vi "OverviewGUI.vi"() -> ()   [LabVIEW 2011]
panel:
  in  "End":bool
  in  "Registerkarte":enum32{"Goto", "Load file", "Load mem", "debug"}(tab)=enum."Load file"
  in  "pos [m]":cluster{dbl, dbl} {"?" format="%#_6p"; "?" format="%#_6p"}
  in  "Goto":bool
  in  "max":cluster{dbl, dbl}={0.066325, 0.044039}
  in  "min":cluster{dbl, dbl}={0.053456, 0.031964}
  in  "Load":bool
  in  "Single tiff":path
  in  "Val2":sgl=4095.0
  in  "Val1":sgl
  in  "Mode":enum16{"Min, Max", "Low%,High%", "Full"}(ring)
  in  "OK-Schaltfläche":bool
  in  "exp.":string="experiment700"
  in  "Pixels":dbl=1000000.0
  in  "Clear":bool
  in  "Add":bool
  in  "Number":u16
  in  "Start":u16
  in  "Calculate":bool
  in  "IMAQs":i32[](array[numeric])
  in  "Transform (Center first)":T1={"Center"={0.0, 0.0}, "Rotate (rad)"=0.0, "MirrorY"=FALSE, "Scale"=1.0}
  out "Image":T2(plugin-control)
  # "known corner coordinates"
  # "left down"
  # "right up"
  # "135CCD"
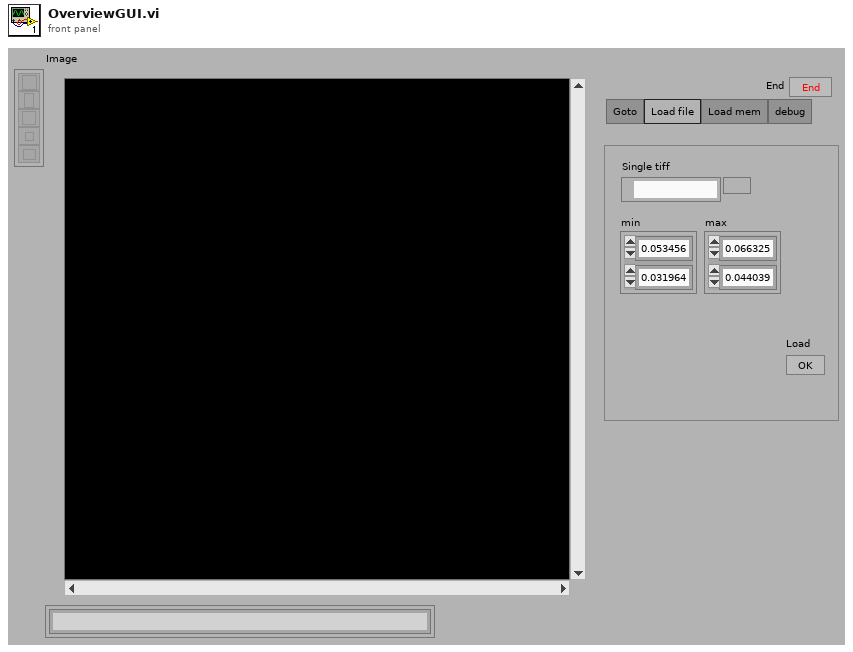
[diagram p1: front panel]
types:
  T1 = cluster{"Center":cluster{dbl, dbl}, "Rotate (rad)":dbl, "MirrorY":bool, "Scale":dbl}
  T2 = typedef "IMAQ Image.ctl" = refnum<image>
  T3 = typedef "Image Type" = u32
  T4 = enum16{"None/#Datasets", "Clear", "TagValueOf#", "AddValues", "ReadValue", "ChangeValue", "Get all"}
  T5 = enum16{"status", "createIMAQ", "getIMAQ", "getNumber", "deleteIMAQ", "deleteAll", "MemoryUsage", "GetAccess", "DecreaseAccess", "ActualIndex", "ElementToNumber"}
  T6 = enum16{"status", "saveMeta", "getMeta", "deleteMeta", "deleteAll", "MemoryUsage"}
  T7 = cluster{"Global Rectangle":i32[], "Contours":cluster{"Contour Type":u32, "ROI Type":u32, "Points":i32[]}[]}
  T8 = typedef "IMAQ Point" = cluster{"X":sgl, "Y":sgl}
  T9 = cluster{cluster{dbl, dbl}, dbl, bool, "pixel/size":dbl}
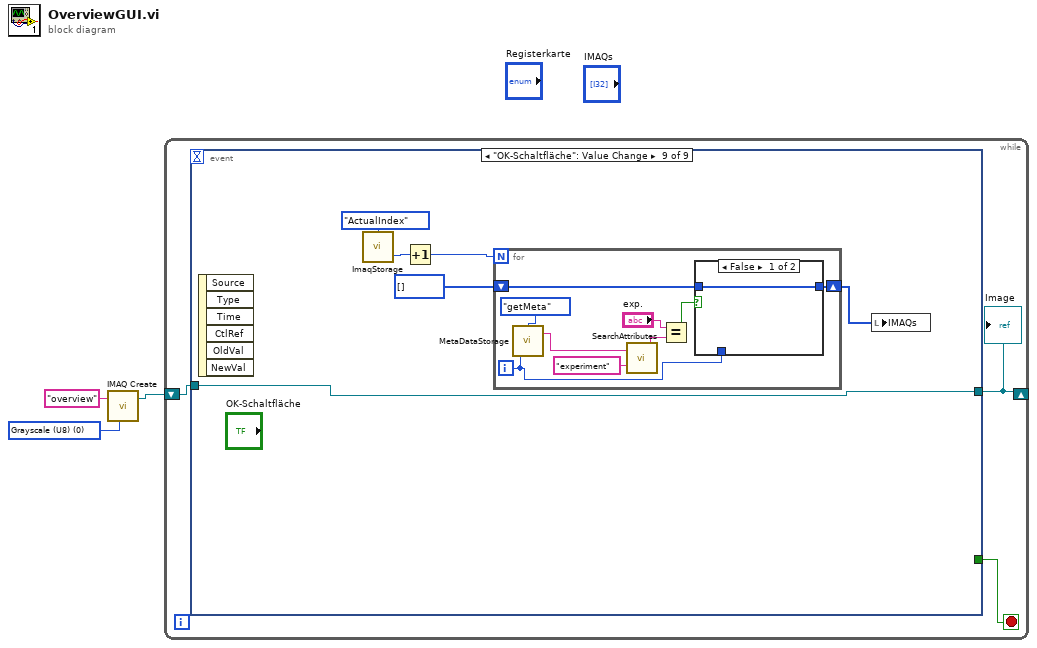
[diagram p0: block diagram]
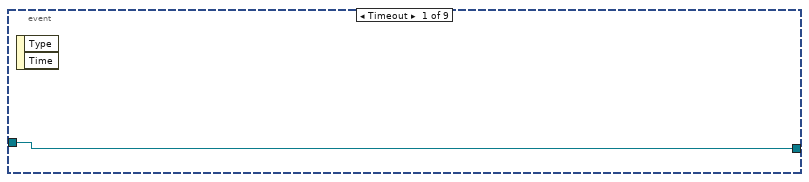
[diagram p2: hidden frame]
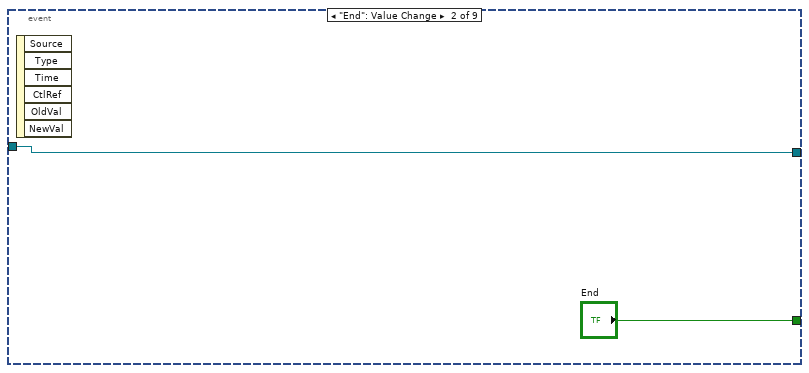
[diagram p3: hidden frame]
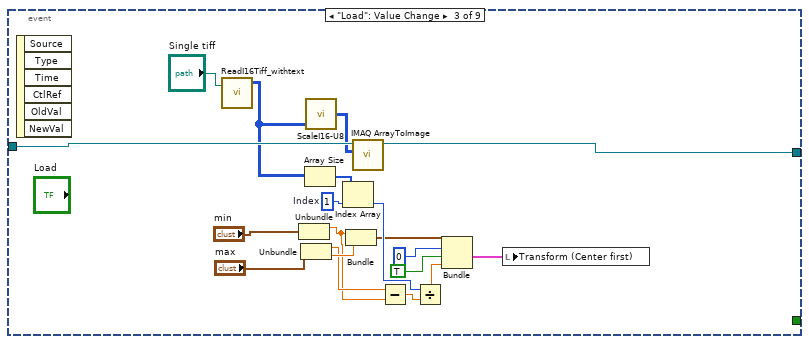
[diagram p4: hidden frame]
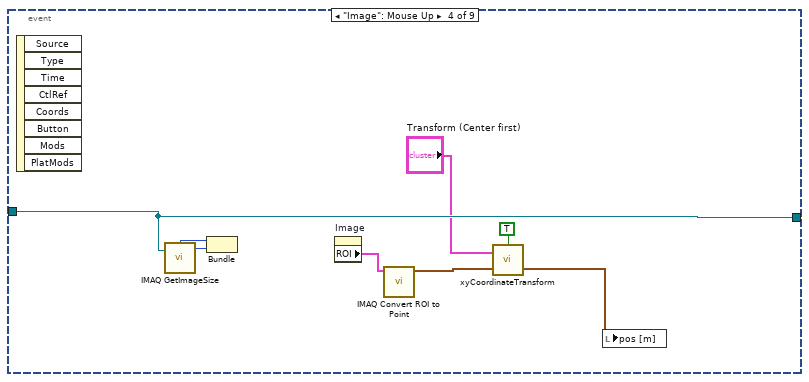
[diagram p5: hidden frame]
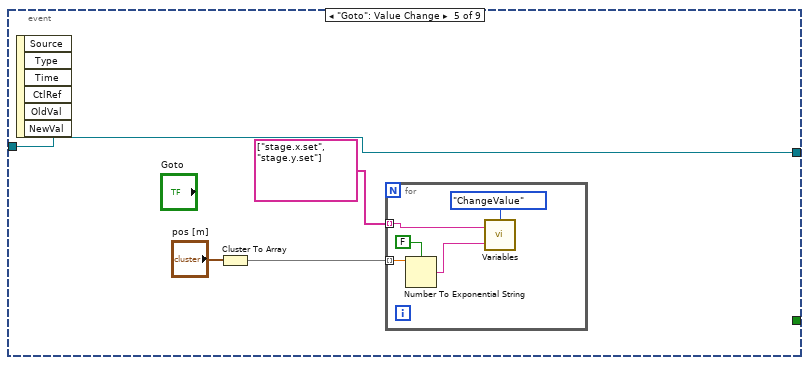
[diagram p6: hidden frame]
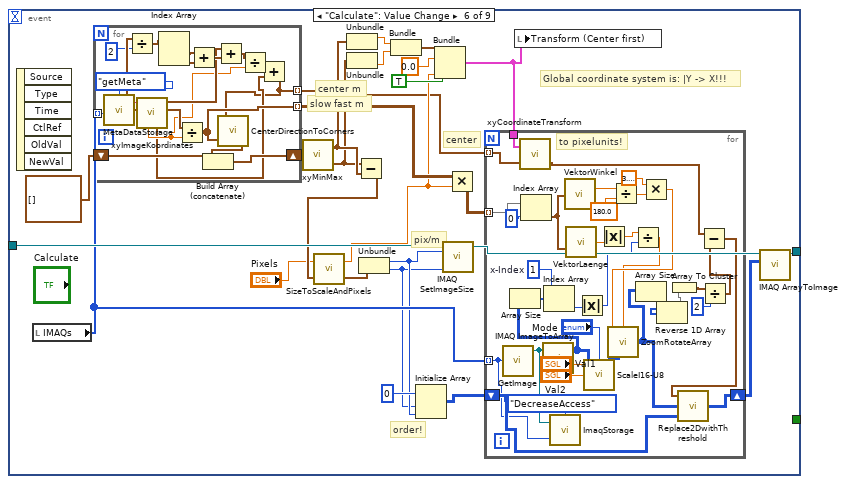
[diagram p7: hidden frame]
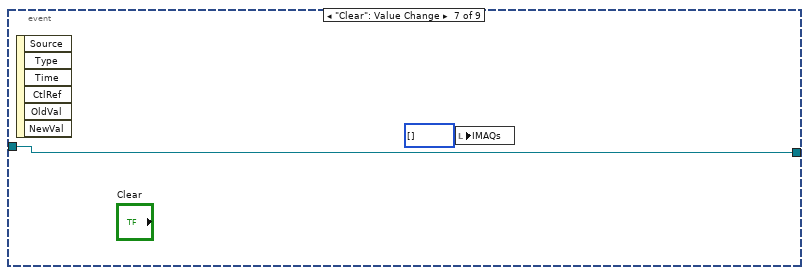
[diagram p8: hidden frame]
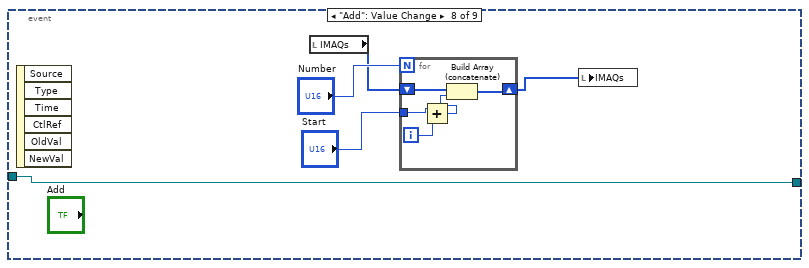
[diagram p9: hidden frame]
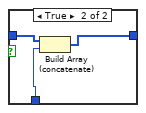
[diagram p10: hidden frame]
diagram:
  w3 = T3 0 items=["Grayscale (U8)", "Grayscale (I16)", "Grayscale (SGL)", "Complex (CSG)", "RGB (U32)", "HSL (U32)", "RGB (U64)"] ("Image Type")
  n1 = call "IMAQ Create"("Image Name"="overview", "Image Type"=w3) -> ("New Image"=w1:T2)  [unwired: 2 in, 2 out]
  n2 = while {
    shift-right: [w4] -> _
    shift-left: w1 -> [w5]
    stop <- w6 stop-if-true
    n3 = event shown="[8] \"OK-Schaltfläche\": Value Change" {
      selector: _ -> [_ _ _ _ _ _ _ _ _]
      dyn-events: _ -> [_ _ _ _ _ _ _ _ _]
      timeout: _ -> [_ _ _ _ _ _ _ _ _]
      tunnel: [_ "End" _ _ _ _ _ _ _] -> w6
      tunnel: w5 -> [w7 w8 w27 w35 w37 w71 w126 w128 w138]
      tunnel: [w7 w8 w26 w35 w37 w65 w126 w128 w138] -> w4
      event Timeout {
        n4 = event-data() -> ()  [unwired: 3 out]
      }
      event "End": Value Change {
        n5 = event-data() -> ()  [unwired: 7 out]
      }
      event "Load": Value Change {
        w14 = 1  # Index
        n6 = event-data() -> ()  [unwired: 7 out]
        n7 = call "ReadI16Tiff_withtext.vi"("file path"="Single tiff") -> ("I16 pixmap"=w16:i16[][])  [unwired: 1 in, 2 out]
        n8 = Unbundle("min") -> (w17:dbl)  [unwired: 1 out]
        n9 = Unbundle("max") -> (w18:dbl, w20:dbl)
        n10 = Array Size(array=w16) -> (size(s)=w15:i32[])
        n11 = call "ScaleI16-U8.vi"("Image I16"=w16) -> ("Image U8"=w25:u8[][])  [unwired: 3 in]
        n12 = Index Array(array=w15, index=w14) -> (element=w13:i32)
        n13 = Bundle(w17, w20) -> (w10:cluster{dbl, dbl})  [unwired: 1 out]
        n14 = call "IMAQ ArrayToImage"("Image Pixels (U8)"=w25, "Image"=w27) -> ("Image Out"=w26:T2)  [unwired: 4 in, 5 out]
        n15 = Subtract(x=w18, y=w17) -> (x-y=w12:dbl)
        n16 = Divide(x=w13, y=w12) -> (x/y=w11:dbl)
        n17 = Bundle(w10, 0, TRUE, w11) -> (w19:cluster{cluster{dbl, dbl}, i32, bool, dbl})  [unwired: 1 out]
        n18 = local write "Transform (Center first)"(w19) -> ()
      }
      event "Image": Mouse Up {
        n19 = event-data() -> ()  [unwired: 9 out]
        n20 = call "IMAQ GetImageSize"("Image"=w35) -> ("Y Resolution"=w33:i32, "X Resolution"=w34:i32)  [unwired: 1 in, 3 out]
        n21 = Bundle("X Resolution"=w34, "Y Resolution"=w33) -> ()  [unwired: 2 out]
        n22 = property on="Image" class="ImageControl"() -> ("ROI"=w36:T7)  [unwired: 2 in, 2 out]
        n23 = call "IMAQ Convert ROI to Point"("ROI Descriptor"=w36) -> ("Point"=w32:T8)  [unwired: 1 in, 8 out]
        n24 = call "xyCoordinateTransform.vi"("Point in"=w32, "Transform (Center first)"="Transform (Center first)", "Back"=TRUE) -> ("Point Out"=w31:cluster{dbl, dbl})  [unwired: 2 out]
        n25 = local write "pos [m]"(w31) -> ()
      }
      event "Goto": Value Change {
        n26 = event-data() -> ()  [unwired: 7 out]
        n27 = Cluster To Array(cluster="pos [m]") -> (array=w39:dbl[])
        n28 = for {
          tunnel: w39 -> [w45] mode=indexing
          tunnel: string[] ["stage.x.set", "stage.y.set"] -> [w42] mode=indexing
          n29 = Number To Exponential String(number=w45, 1:FALSE ("Systemdezimalzeichen verwenden (T)")) -> (E-format string=w41:string)  [unwired: 2 out]
          n30 = call "Variables.vi"("value"=w41, "Tag in"=w42, "Command"=T4."ChangeValue") -> ()  [unwired: 3 out]
        }
      }
      event "Calculate": Value Change {
        # "slow fast m"
        # "center m"
        # "center"
        # "Global coordinate system is: |Y -> X!!!"
        # "order!"
        # "pix/m"
        n31 = event-data() -> ()  [unwired: 7 out]
        n32 = local read "IMAQs"() -> (w68:i32[])
        n33 = for {
          tunnel: w68 -> [w125] mode=indexing
          tunnel: [w107] -> w46 mode=indexing
          tunnel: [w120] -> w70 mode=indexing
          shift-right: [w122] -> w61
          shift-left: cluster{dbl, dbl}[] [] -> [w124]
          n34 = call "MetaDataStorage.vi"("Number"=w125, "Command"=T6."getMeta") -> ("Mata out"=w121:string)  [unwired: 1 in, 1 out]
          n35 = call "xyImageKoordinates.vi"("String"=w121) -> ("fast/slow [m(ii)]"=w118:cluster{"x":dbl, "y":dbl}[], "start [m(ii)] (without stage)"=w112:cluster{dbl, dbl}, "stage [m]"=w108:cluster{dbl, dbl}, "used magnification"=w110:sgl)  [unwired: 5 in, 2 out]
          n36 = Divide(x=w118, y=2) -> (x/y=w116:cluster{"x":dbl, "y":dbl}[])
          n37 = Index Array(array=w116) -> (element #1=w115:cluster{"x":dbl, "y":dbl}, element #2=w114:cluster{"x":dbl, "y":dbl})  [unwired: 2 in]
          n38 = Divide(x=w118, y=w110) -> (x/y=w120:cluster{"x":dbl, "y":dbl}[])
          n39 = Add(x=w115, y=w114) -> (x+y=w113:cluster{"x":dbl, "y":dbl})
          n40 = Add(x=w112, y=w113) -> (x+y=w111:cluster{dbl, dbl})
          n41 = Divide(x=w111, y=w110) -> (x/y=w109:cluster{dbl, dbl})
          n42 = Add(x=w109, y=w108) -> (x+y=w107:cluster{dbl, dbl})
          n43 = call "CenterDirectionToCorners.vi"("Fast/Slow"=w120, "Center"=w107) -> ("AllCorners"=w123:cluster{dbl, dbl}[])
          n44 = Build Array (concatenate)(w124, w123) -> (w122:cluster{dbl, dbl}[])
        }
        n45 = call "xyMinMax.vi"("XY Graph"=w61) -> ("min"=w55:cluster{dbl, dbl}, "max"=w54:cluster{dbl, dbl})
        n46 = Unbundle(w55) -> (w52:dbl)  [unwired: 1 out]
        n47 = Unbundle(w54) -> (w51:dbl)  [unwired: 1 out]
        n48 = Subtract(x=w54, y=w55) -> (x-y=w60:cluster{dbl, dbl})
        n49 = call "SizeToScaleAndPixels.vi"("size"=w60, "Pixels"="Pixels") -> ("Pixels"=w59:cluster{"pixelsx":i32, "pixelsy":i32}, "pixel/size"=w48:dbl)
        n50 = Unbundle(w59) -> ("pixelsx"=w57:i32, "pixelsy"=w56:i32)
        n51 = Bundle(w52, w51) -> (w53:cluster{dbl, dbl})  [unwired: 1 out]
        n52 = Initialize Array(u8 0, w56, w57) -> (w66:u8[][])
        n53 = Bundle(w53, 0.0, TRUE, "pixel/size"=w48) -> (w47:T9)  [unwired: 1 out]
        n54 = call "IMAQ SetImageSize"("Y Resolution"=w56, "X Resolution"=w57, "Image"=w71) -> ("Image Out"=w64:T2)  [unwired: 1 in, 2 out]
        n55 = Multiply(x=w70, y=w48) -> (x*y=w69:cluster{"x":dbl, "y":dbl}[][])
        n56 = for {
          tunnel: w69 -> [w102] mode=indexing
          tunnel: w68 -> [w80] mode=indexing
          shift-right: [w85] -> w63
          shift-left: w66 -> [w89]
          tunnel: w47 -> [w74]
          tunnel: w46 -> [w73] mode=indexing
          w105 = 1  # x-Index
          # "to pixelunits!"
          n57 = call "GetImage.vi"("Image Number"=w80) -> ("Image"=w83:T2)  [unwired: 3 out]
          n58 = call "xyCoordinateTransform.vi"("Point in"=w73, "Transform (Center first)"=w74) -> ("Point Out"=w72:cluster{dbl, dbl})  [unwired: 1 in, 2 out]
          n59 = Index Array(array=w102, index=0 ("Index")) -> (element=w97:cluster{"x":dbl, "y":dbl})
          n60 = call "IMAQ ImageToArray"("Image"=w83) -> ("Image Pixels (I16)"=w82:i16[][])  [unwired: 2 in, 5 out]
          n61 = Array Size(array=w82) -> (size(s)=w106:i32[])
          n62 = Index Array(array=w106, index=w105) -> (element=w101:i32)
          n63 = call "ImaqStorage.vi"("Number"=w80, "IMAQ in"=w83, "Command"=T5."DecreaseAccess") -> ()  [unwired: 2 out]
          n64 = call "VektorWinkel.vi"("Vektor"=w97) -> ("Vektorwinkel [degrees]"=w100:dbl)
          n65 = call "VektorLaenge.vi"("Vektor"=w97) -> ("Vektorlänge"=w104:dbl)
          n66 = Absolute Value(x=w101) -> (abs(x)=w86:i32)
          n67 = call "ScaleI16-U8.vi"("Mode"="Mode", "Image I16"=w82, "Val2"="Val2", "Val1"="Val1") -> ("Image U8"=w90:u8[][])
          n68 = Absolute Value(x=w104) -> (abs(x)=w87:dbl)
          n69 = Divide(x=w100, y=180.0) -> (x/y=w99:dbl)
          n70 = Divide(x=w87, y=w86) -> (x/y=w94:dbl)
          n71 = Multiply(x=3.141592653589793, y=w99) -> (x*y=w95:dbl)
          n72 = call "ZoomRotateArray.vi"("Zoom"=w94, "Image"=w90, "Angle [rad]"=w95) -> ("Intensitätsgraph"=w88:u8[][])
          n73 = Array Size(array=w88) -> (size(s)=w76:i32[])
          n74 = Reverse 1D Array(array=w76) -> (reversed array=w75:i32[])
          n75 = Array To Cluster(array=w75) -> (cluster=w93:cluster{"[0]":i32, "[1]":i32})
          n76 = Divide(x=w93, y=2) -> (x/y=w91:cluster{"[0]":dbl, "[1]":dbl})
          n77 = Subtract(x=w72, y=w91) -> (x-y=w84:cluster{dbl, dbl})
          n78 = call "Replace2DwithThreshold.vi"("Array in"=w89, "replace part"=w88, "replace position"=w84) -> ("Array Out"=w85:u8[][])
        }
        n79 = local write "Transform (Center first)"(w47) -> ()
        n80 = call "IMAQ ArrayToImage"("Image Pixels (U8)"=w63, "Image"=w64) -> ("Image Out"=w65:T2)  [unwired: 4 in, 5 out]
      }
      event "Clear": Value Change {
        n81 = event-data() -> ()  [unwired: 7 out]
        n82 = local write "IMAQs"(i32[] [] ("IMAQs")) -> ()
      }
      event "Add": Value Change {
        n83 = event-data() -> ()  [unwired: 7 out]
        n84 = local read "IMAQs"() -> (w131:i32[])
        n85 = for {
          N: "Number" -> [_]
          shift-right: [w136] -> w129
          shift-left: w131 -> [w137]
          tunnel: "Start" -> [w135]
          i -> [w134]
          n86 = Add(x=w135, y=w134) -> (x+y=w133:i32)
          n87 = Build Array (concatenate)(w137, w133) -> (w136:i32[])
        }
        n88 = local write "IMAQs"(w129) -> ()
      }
      event "OK-Schaltfläche": Value Change {
        n89 = event-data() -> ()  [unwired: 7 out]
        n90 = call "ImaqStorage.vi"("Command"=T5."ActualIndex") -> ("Number out"=w141:i32)  [unwired: 2 in, 1 out]
        n91 = Increment(x=w141) -> (x+1=w142:i32)
        n92 = for {
          N: w142 -> [_]
          shift-right: [w145] -> w140
          shift-left: i32[] [] -> [w144]
          i -> [w146]
          n93 = call "MetaDataStorage.vi"("Number"=w146, "Command"=T6."getMeta") -> ("Mata out"=w150:string)  [unwired: 1 in, 1 out]
          n94 = call "SearchAttributes.vi"("Search"="experiment", "String"=w150) -> ("ValueText"=w148:string)
          n95 = Equal?(x="exp.", y=w148) -> (x = y?=w147:bool)
          n96 = case shown="False" w147 {
            tunnel: w146 -> [_ w156]
            tunnel: [w153 w155] -> w145
            tunnel: w144 -> [w153 w154]
            frame False {
            }
            frame True {
              n97 = Build Array (concatenate)(w154, w156) -> (w155:i32[])
            }
          }
        }
        n98 = local write "IMAQs"(w140) -> ()
      }
    }
    "Image" <- w4
  }
